vi "_IMPLEMENT_.vi"(0 "VI Refnum":refnum<vi>, 1 "Dialog (T)":bool=TRUE, 2 "Message":string, 3 "error in (no error)":errorcluster, 4 "Function Name":string) -> (10 "error out":errorcluster)   [LabVIEW 2025]
doc: "This VI inserts a \"not implemented\" warning or error into the error cluster."
uses:
  <vilib>/Utility/miscctls.llb/LVPointTypeDef.ctl
  Application/App_Support.llb/App_Support.lvlib
panel:
  in  "About":bool
  in  "Save":bool
  in  "Open VI":bool
  out "scrollbar text":string
  in  "OK":bool
  in  "Cancel":bool
  out "Source of Error":string="#IMPLEMENTATION - Function yet not implemented :-O"
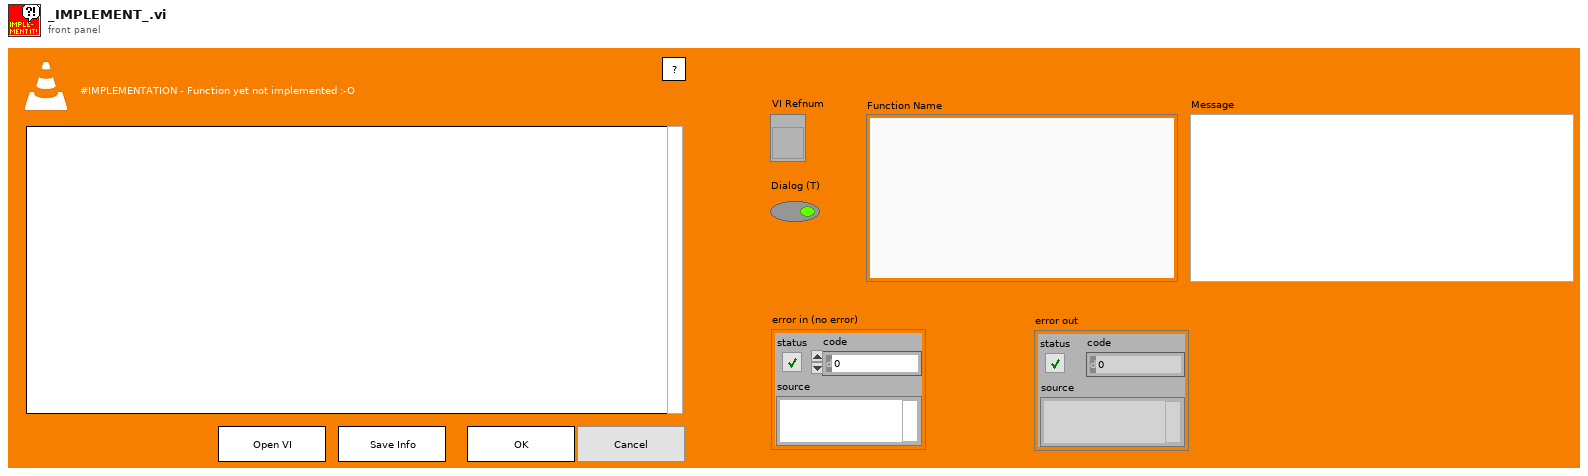
[diagram p1: front panel]
types:
  T1 = typedef "LVPointTypeDef.ctl" = cluster{"Horizontal":i16, "Vertical":i16}
  T2 = enum32{"invalid VI type", "Standard VI", "Control VI", "Global VI", "Polymorphic VI", "Configuration VI", "SubSystem", "Facade VI", "Method VI", "Statechart Diagram VI"}
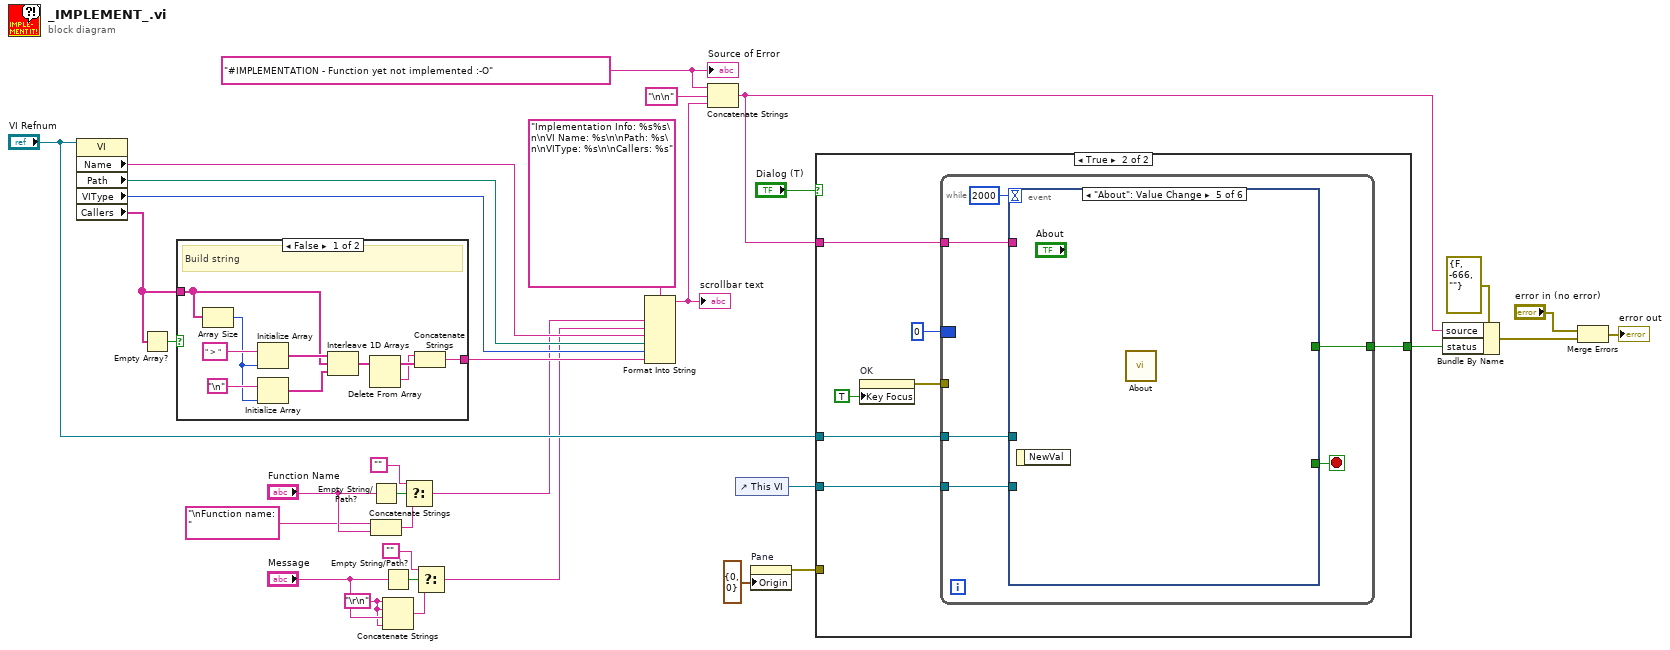
[diagram p0: block diagram]
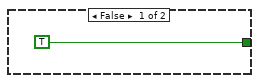
[diagram p2: hidden frame]
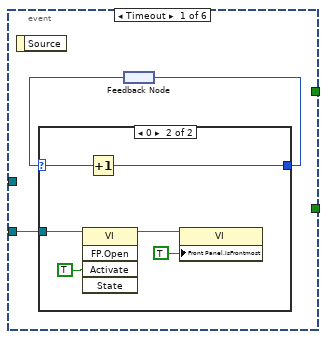
[diagram p3: hidden frame]
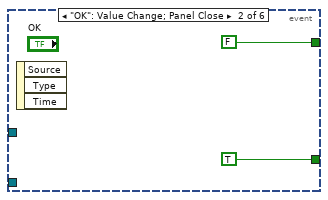
[diagram p5: hidden frame]
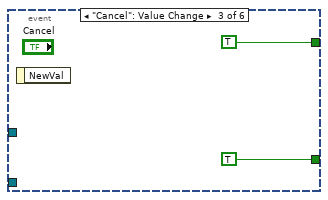
[diagram p6: hidden frame]
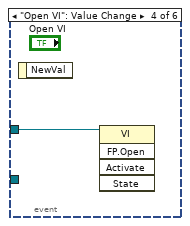
[diagram p7: hidden frame]
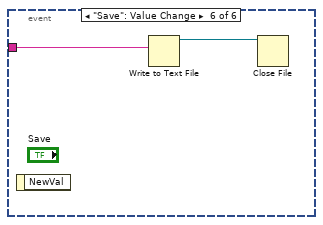
[diagram p8: hidden frame]
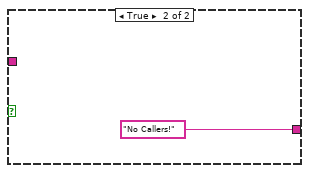
[diagram p9: hidden frame]
diagram:
  w1 = "\r\n"
  w17 = "#IMPLEMENTATION - Function yet not implemented :-O" ("source")
  n1 = property class="VI"(reference="VI Refnum") -> ("Name"=w16:string, "Path"=w24:path, "VIType"=w25:T2, "Callers"=w30:string[])  [unwired: 1 in, 2 out]
  n2 = Empty Array?(array=w30) -> (empty?=w31:bool)
  n3 = case shown="False" w31 {
    tunnel: w30 -> [w39 _]
    tunnel: [w37 "No Callers!"] -> w26
    frame False {
      # "Build string"
      n4 = Array Size(array=w39) -> (size(s)=w41:i32)
      n5 = Initialize Array(" > ", w41) -> (w40:string[])
      n6 = Initialize Array("\n", w41) -> (w38:string[])
      n7 = Interleave 1D Arrays(w40, w39, w38) -> (w36:string[])
      n8 = Delete From Array(array=w36) -> (deleted portion=w34:string, array with subset deleted=w35:string[])  [unwired: 2 in]
      n9 = Concatenate Strings(w34, w35) -> (w37:string)
    }
    frame True {
    }
  }
  n10 = Empty String/Path?(string/path="Function Name") -> (empty?=w12:bool)
  n11 = Concatenate Strings("\nFunction name: " ("string"), "Function Name") -> (w9:string)
  n12 = Empty String/Path?(string/path="Message") -> (empty?=w5:bool)
  n13 = Concatenate Strings(w1, w1, "Message", w1) -> (w7:string)
  n14 = Select(t="", s=w12, f=w9) -> (s? t:f=w8:string)
  n15 = Select(t="", s=w5, f=w7) -> (s? t:f=w3:string)
  n16 = Format Into String(format string="Implementation Info: %s%s\n\nVI Name: %s\n\nPath: %s\n\nVIType: %s\n\nCallers: %s" ("source"), w8, w3, w16, w24, w25, w26) -> (resulting string=w22:string)  [unwired: 2 in, 1 out]
  "scrollbar text" <- w22
  n17 = Concatenate Strings(w17, "\n\n" ("string"), w22) -> (w18:string)
  n18 = control-ref of="This VI"() -> (w13:refnum<vi>)
  n19 = property on="Pane" class="Pane"("Origin"=T1 {"Horizontal"=0, "Vertical"=0}) -> (error out=w14:errorcluster)  [unwired: 2 in, 1 out]
  n20 = case shown="True" "Dialog (T)" {
    tunnel: "VI Refnum" -> [_ w52]
    tunnel: [TRUE w51] -> w20
    tunnel: w18 -> [_ w48]
    tunnel: w14 -> [_ _]
    tunnel: w13 -> [_ w46]
    frame False {
    }
    frame True {
      n21 = property on="OK" class="Bool"("Key Focus"=TRUE) -> (error out=w50:errorcluster)  [unwired: 2 in, 1 out]
      n22 = while {
        tunnel: w52 -> [w58]
        tunnel: [w57] -> w51
        tunnel: w50 -> [_]
        tunnel: w48 -> [w55]
        border: 0 -> [_]
        tunnel: w46 -> [w53]
        stop <- w56 stop-if-true
        n23 = event shown="[4] \"About\": Value Change" {
          selector: _ -> [_ _ _ _ _ _]
          dyn-events: _ -> [_ _ _ _ _ _]
          timeout: 2000 -> [_ _ _ _ _ _]
          tunnel: w58 -> [_ _ _ w73 _ _]
          tunnel: [_ FALSE TRUE _ _ _] -> w57
          tunnel: [_ TRUE TRUE _ _ _] -> w56
          tunnel: w55 -> [_ _ _ _ _ w75]
          tunnel: w53 -> [w59 _ _ _ _ _]
          event Timeout {
            n24 = event-data() -> ()  [unwired: 1 in, 1 out]
            n25 = feedback #1() -> (w61:i32)
            n26 = case shown="0" w61 {
              selector: w61 -> [w62 w67]
              tunnel: [w62 w66] -> w60
              tunnel: w59 -> [_ w63]
              frame Default {
              }
              frame 0 {
                n27 = invoke class="VI" method="FP.Open"(reference=w63, "Activate"=TRUE ("Activate?")) -> (reference out=w65:refnum<vi>)  [unwired: 3 in, 4 out]
                n28 = Increment(x=w67) -> (x+1=w66:i32)
                n29 = property class="VI"(reference=w65, "Front Panel.IsFrontmost"=TRUE ("Front Panel Window:Is Frontmost")) -> ()  [unwired: 1 in, 2 out]
              }
            }
            n30 = feedback-in #1(w60) -> ()
          }
          event "OK": Value Change; Panel Close {
            n31 = event-data() -> ()  [unwired: 1 in, 3 out]
          }
          event "Cancel": Value Change {
            n32 = event-data() -> ()  [unwired: 1 in, 1 out]
          }
          event "Open VI": Value Change {
            n33 = event-data() -> ()  [unwired: 1 in, 1 out]
            n34 = invoke class="VI" method="FP.Open"(reference=w73) -> ()  [unwired: 4 in, 5 out]
          }
          event "About": Value Change {
            n35 = event-data() -> ()  [unwired: 1 in, 1 out]
            n36 = call "About.vi"() -> ()  [unwired: 11 in, 1 out]
          }
          event "Save": Value Change {
            n37 = event-data() -> ()  [unwired: 1 in, 1 out]
            n38 = Write to Text File(text=w75) -> (refnum out=w74:refnum<file>)  [unwired: 3 in, 2 out]
            n39 = Close File(refnum=w74) -> ()  [unwired: 1 in, 2 out]
          }
        }
      }
    }
  }
  n40 = Bundle By Name(cluster=errorcluster {"status"=FALSE, "code"=-666, "source"=""} ("error out"), "source"=w18, "status"=w20) -> (w28:errorcluster)
  n41 = Merge Errors("error in (no error)", w28) -> (→"error out":errorcluster)
  "Source of Error" <- w17
